vi "Write Spectrum Notifier.vi"(8 "error in (no error)":errorcluster, 11 "Waveform":waveform(dbl)) -> (0 "error out":errorcluster)   [LabVIEW 2017]
uses:
  Application Control/Application Globals.vi
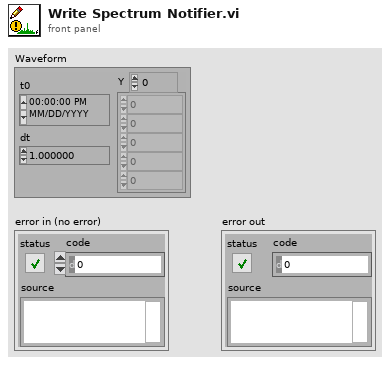
[diagram p1: front panel]
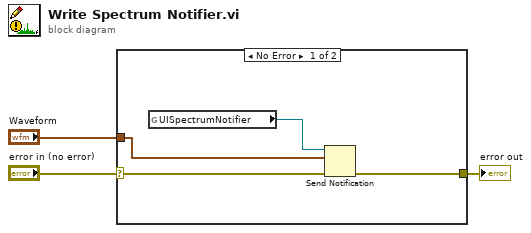
[diagram p0: block diagram]
diagram:
  n1 = case shown="No Error" "error in (no error)" {
    selector: "error in (no error)" -> [w4 w8]
    tunnel: [w7 w8] -> w1
    tunnel: "Waveform" -> [w5 _]
    frame No Error {
      n2 = global read "Application Globals.vi" "UISpectrumNotifier"() -> (w6:refnum<notifier>)
      n3 = Send Notification(notification=w5, notifier=w6, error in (no error)=w4) -> (error out=w7:errorcluster)  [unwired: 1 out]
    }
    frame Error {
    }
  }
  "error out" <- w1
